vi "Do.vi"(8 "error in (no error)":errorcluster, 10 "Actor in":refnum<class "Actor.lvclass">, 11 "Update Humidifier Controller MSG":refnum<class "Update Humidifier Controller MSG.lvclass">) -> (0 "error out":errorcluster, 2 "Actor out":refnum<class "Actor.lvclass">)   [LabVIEW 2014, in "Humidifier Test Lib.lvlib" / "Update Humidifier Controller MSG.lvclass"]
doc: "(<B>Filename</B>: Actor Framework.lvlib:Message.lvclass:Do.vi)\n\nDefines what a message does when it is received by an actor. Generally, a message instructs an actor to invoke one of its methods. By default, this method does nothing. A child class must override it to define behavior. Create a child class by using the Actor Framework Message Maker dialog box."
uses:
  Update Humidifier Controller MSG.lvclass
  <vilib>/ActorFramework/Actor/Actor.lvclass
  TEC Controller.lvclass
  reusable/DAQ Device/Device/Generic Data Update Data MSG/Generic Update Data Message.lvclass/Generic Update Data Message.ctl
  Devices/Meerstetter TEC/Data/mTEC Data.lvclass
  TEC Controller.lvclass/TEC Controller.ctl
  Devices/Meerstetter TEC/Data/mTEC Data.lvclass/mTEC Data.ctl
  Devices/Vaisala Probe/Data/Vaisala Data.lvclass
  Devices/Vaisala Probe/Data/Vaisala Data.lvclass/Vaisala Data.ctl
  Devices/Alicat/Session Based/Data/Alicat Data.lvclass
  Devices/Alicat/Session Based/Data/Alicat Data.lvclass/Alicat Data.ctl
  Read TEC.vi
  Devices/Meerstetter TEC/Data/Read Tobj.vi
  Devices/Meerstetter TEC/Data/Read Vout.vi
  Devices/Vaisala Probe/Data/Read T.vi
  Devices/Vaisala Probe/Data/Read Td.vi
  Devices/Vaisala Probe/Data/Read RH.vi
  Read Vaisala.vi
  Devices/Alicat/Session Based/Data/Accessors/Read Data.vi
  Read Alicat.vi
  reusable/DAQ Device/Device/Generic Data Update Data MSG/Read ID.vi
  reusable/DAQ Device/Device/Generic Data Update Data MSG/Read Data.vi
  reusable/Data/Data.lvclass
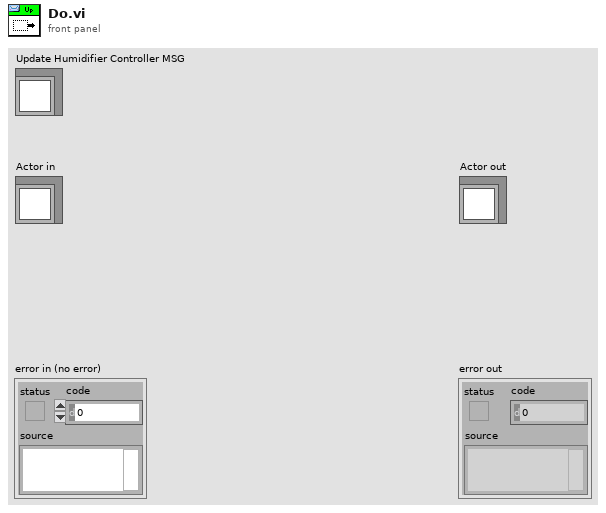
[diagram p1: front panel]
types:
  T1 = cluster{"T (degC)":dbl, "Td (degC)":dbl, "RH (%)":dbl}
  T2 = cluster{"T":dbl, "P":dbl, "Q":dbl, "Q0":dbl, "Qsp":dbl}
  T3 = cluster{"P":sgl, "T":sgl, "Q":sgl, "Qsp":sgl, "Q0":sgl}
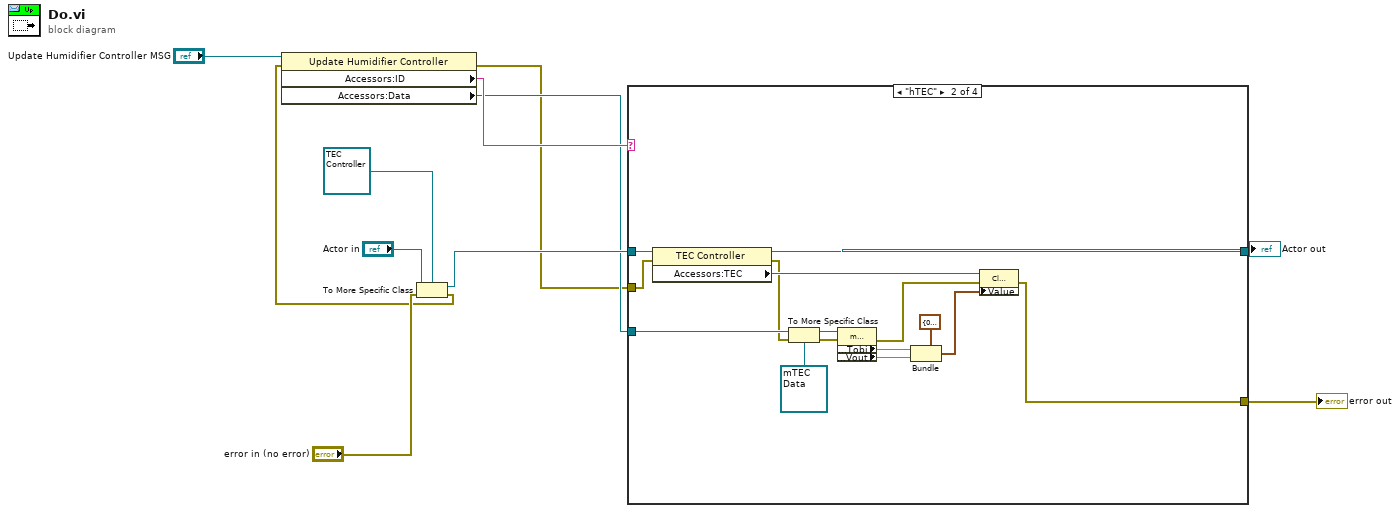
[diagram p0: block diagram]
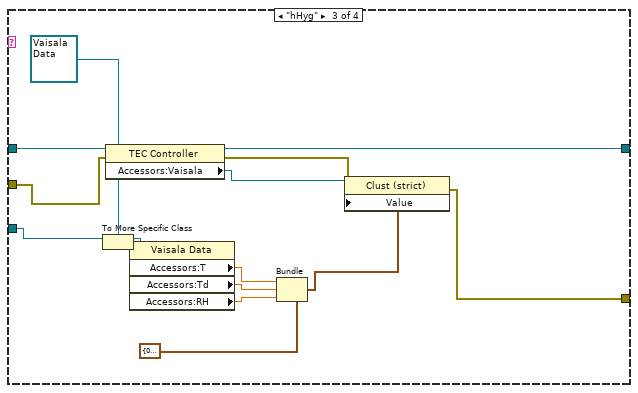
[diagram p3: hidden frame]
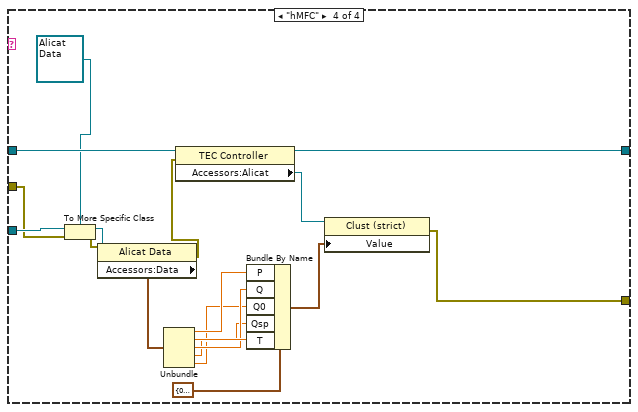
[diagram p4: hidden frame]
diagram:
  n1 = To More Specific Class(target class=refnum<class "TEC Controller.lvclass"> refnum ("Humidifier Test Lib.lvlib:TEC Controller"), reference="Actor in", error in="error in (no error)") -> (specific class reference=w6:refnum<class "TEC Controller.lvclass">, error out=w2:errorcluster)
  n2 = property class="Update Humidifier Controller"(reference="Update Humidifier Controller MSG", error in=w2) -> (error out=w1:errorcluster, "Accessors:ID"=w7:string, "Accessors:Data"=w4:refnum<class "Data.lvclass">)  [unwired: 1 out]
  n3 = case shown="\"hTEC\"" w7 {
    tunnel: w6 -> [w13 w28 w40 w56]
    tunnel: [w13 w26 w31 w55] -> w5
    tunnel: w1 -> [w12 w27 w29 w59]
    tunnel: w4 -> [_ w25 w42 w60]
    tunnel: [w12 w14 w32 w50] -> w3
    frame "Null", Default {
    }
    frame "hTEC" {
      n4 = property class="TEC Controller"(reference=w28, error in=w27) -> (reference out=w26:refnum<class "TEC Controller.lvclass">, error out=w17:errorcluster, "Accessors:TEC"=w23:refnum<vi>)
      n5 = To More Specific Class(target class=refnum<class "mTEC Data.lvclass"> refnum ("Meerstetter Lib.lvlib:mTEC Data.lvclass"), reference=w25, error in=w17) -> (specific class reference=w22:refnum<class "mTEC Data.lvclass">, error out=w16:errorcluster)
      n6 = property class="mTEC Data.lvclass"(reference=w22, error in=w16) -> (error out=w15:errorcluster, "Accessors:Tobj"=w20:dbl, "Accessors:Vout"=w19:dbl)  [unwired: 1 out]
      n7 = Bundle(cluster=cluster{"T (degC)":dbl, "Td (degC)":dbl} {"T (degC)"=0.0, "Td (degC)"=0.0} ("Value"), "T (degC)"=w20, "Td (degC)"=w19) -> (w18:cluster{"T (degC)":dbl, "Td (degC)":dbl})
      n8 = property class="Clust (strict)"(reference=w23, error in=w15, "Value"=w18) -> (error out=w14:errorcluster)  [unwired: 1 out]
    }
    frame "hHyg" {
      n9 = To More Specific Class(target class=refnum<class "Vaisala Data.lvclass"> refnum ("Vaisala Library.lvlib:Vaisala Data"), reference=w42) -> (specific class reference=w38:refnum<class "Vaisala Data.lvclass">)  [unwired: 1 in, 1 out]
      n10 = property class="TEC Controller"(reference=w40, error in=w29) -> (reference out=w31:refnum<class "TEC Controller.lvclass">, error out=w30:errorcluster, "Accessors:Vaisala"=w39:refnum<vi>)
      n11 = property class="Vaisala Data"(reference=w38) -> ("Accessors:T"=w37:dbl, "Accessors:Td"=w36:dbl, "Accessors:RH"=w35:dbl)  [unwired: 1 in, 2 out]
      n12 = Bundle(cluster=T1 {"T (degC)"=0.0, "Td (degC)"=0.0, "RH (%)"=0.0} ("Value"), "T (degC)"=w37, "Td (degC)"=w36, "RH (%)"=w35) -> (w33:T1)
      n13 = property class="Clust (strict)"(reference=w39, error in=w30, "Value"=w33) -> (error out=w32:errorcluster)  [unwired: 1 out]
    }
    frame "hMFC" {
      n14 = To More Specific Class(target class=refnum<class "Alicat Data.lvclass"> refnum ("Alicat Lib.lvlib:Alicat Data"), reference=w60, error in=w59) -> (specific class reference=w58:refnum<class "Alicat Data.lvclass">, error out=w57:errorcluster)
      n15 = property class="Alicat Data"(reference=w58, error in=w57) -> (error out=w54:errorcluster, "Accessors:Data"=w48:T3)  [unwired: 1 out]
      n16 = Unbundle(w48) -> ("P"=w47:sgl, "T"=w46:sgl, "Q"=w45:sgl, "Qsp"=w44:sgl, "Q0"=w43:sgl)
      n17 = property class="TEC Controller"(reference=w56, error in=w54) -> (reference out=w55:refnum<class "TEC Controller.lvclass">, "Accessors:Alicat"=w53:refnum<vi>)  [unwired: 1 out]
      n18 = Bundle By Name(cluster=T2 {"T"=0.0, "P"=0.0, "Q"=0.0, "Q0"=0.0, "Qsp"=0.0} ("Value"), "P"=w47, "Q"=w45, "Q0"=w43, "Qsp"=w44, "T"=w46) -> (w51:T2)
      n19 = property class="Clust (strict)"(reference=w53, "Value"=w51) -> (error out=w50:errorcluster)  [unwired: 1 in, 1 out]
    }
  }
  "error out" <- w3
  "Actor out" <- w5
